vi "Enqueue.vi"(7 "Priority (F)":bool, 8 "ErrorArray":errorcluster[](array[cluster]), 9 "Message Data":variant, 10 "Message":string) -> (0 "ErrorArray":errorcluster[](array[cluster]))   [LabVIEW 2014, in "Queue.lvlib"]
uses:
  Queue.lvlib
  clMessage.ctl
  <userlib>/NIST/NISTErrorLib/NISTErrorLib.lvlib
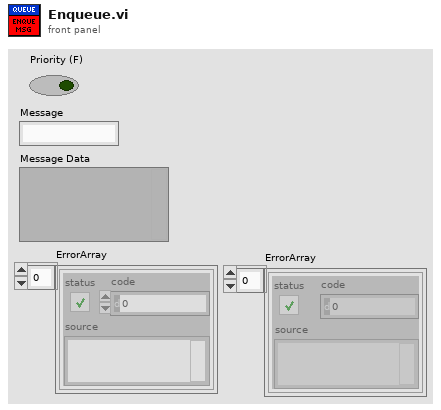
[diagram p1: front panel]
types:
  T1 = typedef "Queue.lvlib/clMessage.ctl" = cluster{"Message":string, "Message Data":variant}
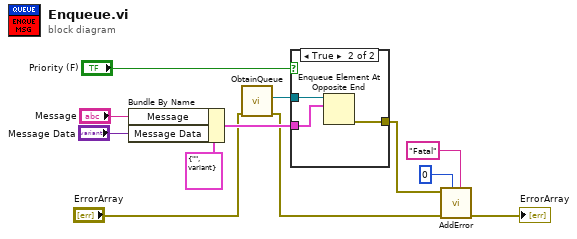
[diagram p0: block diagram]
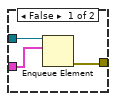
[diagram p2: hidden frame]
diagram:
  n1 = Bundle By Name(cluster=T1 {"Message"="", "Message Data"=variant} ("clMessage"), "Message"="Message", "Message Data"="Message Data") -> (w11:T1)
  n2 = call "ObtainQueue.vi"("ErrorArray"="ErrorArray") -> ("ErrorArray"=w1:errorcluster[], "QueueRef"=w3:refnum<queue>)  [unwired: 9 in]
  n3 = case shown="True" "Priority (F)" {
    tunnel: w11 -> [w14 w18]
    tunnel: w3 -> [w15 w17]
    tunnel: [w13 w16] -> w6
    frame False {
      n4 = Enqueue Element(queue=w15, element=w14) -> (error out=w13:errorcluster)  [unwired: 2 in, 2 out]
    }
    frame True {
      n5 = Enqueue Element At Opposite End(queue=w17, element=w18) -> (error out=w16:errorcluster)  [unwired: 2 in, 2 out]
    }
  }
  n6 = call <userlib>:"AddError.vi"("Severity"="Fatal", "Priority"=u8 0, "ErrorArray"=w1, "error in (no error)"=w6) -> ("ErrorArray"=→"ErrorArray":errorcluster[])  [unwired: 6 in, 1 out]
